vi "FPGA_init_FTL.vi"(6 "queue FPGA IN":refnum<queue>, 7 "FPGA VI Reference in":refnum<k20>, 8 "error in":errorcluster, 10 "variant":variant, 11 "Measuring QPD":bool) -> (0 "error out":errorcluster, 4 "queue FPGA OUT":refnum<queue>, 5 "FPGA VI Reference Out":refnum<k20>)   [LabVIEW 2015]
uses:
  CONTROLS/Q_FPGA_element.ctl
  <vilib>/FPGAPlugInAG/Dynamic/niLvFpga_Reset_Dynamic.vi
  <vilib>/FPGAPlugInAG/Dynamic/niLvFpga_Close_Dynamic.vi
  <vilib>/FPGAPlugInAG/PCIe-7841R/niLvFpga_Open_PCIe-7841R.vi
  <vilib>/rvi/interface/common/dynamic/niFpgaDynamicAddResources.vi
  <vilib>/Utility/error.llb/Error Cluster From Error Code.vi
  <vilib>/rvi/errors/niLvFpgaAdjustHostInterfaceError.vi
  <vilib>/FPGAPlugInAG/Dynamic/niLvFpga_Run_Dynamic.vi
  GLOBAL/Global_FPGA.vi
  <vilib>/rvi/interface/nirviMethod/nirviMethod.xnode
  <vilib>/rvi/interface/nirviCloseFPGA/nirviCloseFPGA.xnode
  <vilib>/rvi/interface/nirviOpenFPGA/nirviOpenFPGA.xnode
  FPGA/FPGA Bitfiles/FPGAv0_FPGATarget_FPGAtriggercamer_zs8MuLZc0ko.lvbitx
  <vilib>/rvi/interface/nirviReadWriteControl/nirviReadWriteControl.xnode
  NiFpgaLv.dll
  <vilib>/rvi/interface/Simulation/niFpgaSimulationCallBeginRW.vi
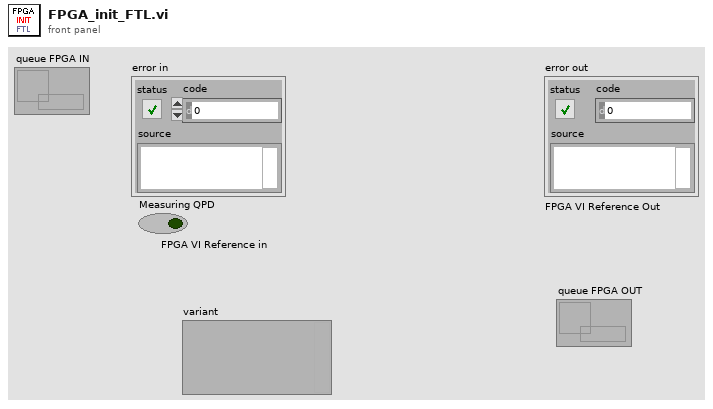
[diagram p1: front panel]
types:
  T1 = typedef "Q_FPGA_element.ctl" = cluster{"variant":variant, "Instruction":enum16{"FPGA_idle", "FPGA_initialize", "FPGA_error", "FPGA_security_stop", "FPGA_laser", "FPGA_start_stop_measure_QPD", "FPGA_measure_QPD", "FPGA_measure_QPD_noise", "FPGA_change_QPD_display", "FPGA_stop_measure_QPD", "FPGA_init_autofocus", "FPGA_init_single_scan", "FPGA_stop_single_scan", "FPGA_init_TL", "FPGA_close_TL", "FPGA_measure_QPD_FTL", "FPGA_init_FTL", "FPGA_init_single_scan_FTL", "FPGA_close_FTL", "FPGA_stop"}}
  T2 = cluster{"N laser lines":i32, "N Z positions":i32, "Laser lines":i32[], "Laser power":sgl[]}
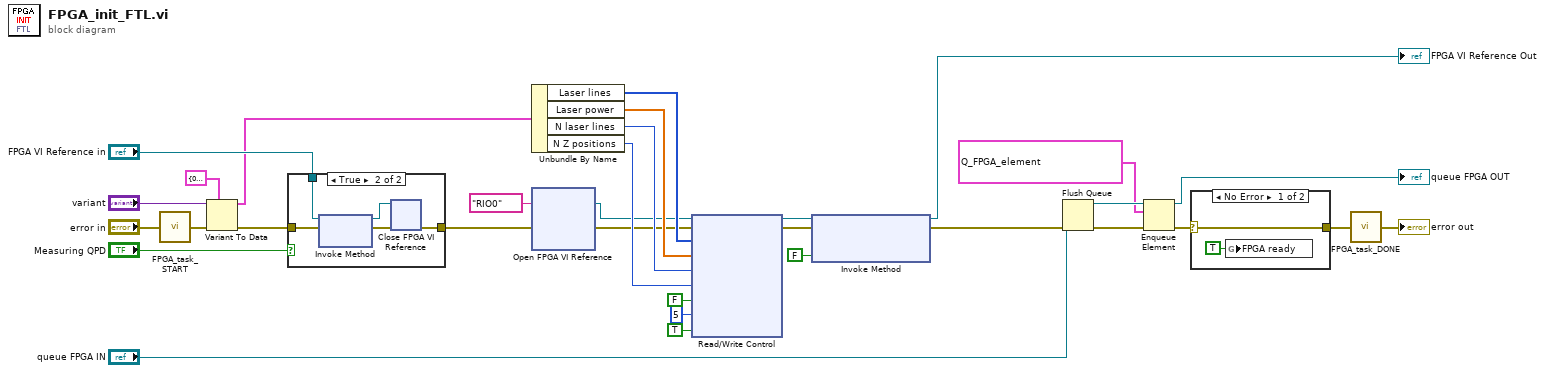
[diagram p0: block diagram]
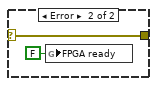
[diagram p3: hidden frame]
diagram:
  n1 = call "FPGA_task_START.vi"("error in"="error in") -> ("error out"=w20:errorcluster)
  n2 = Variant To Data(error in=w20, type=T2 {"N laser lines"=0, "N Z positions"=0, "Laser lines"=[0, 0, 0, 0, 0], "Laser power"=[0.0, 0.0, 0.0, 0.0, 0.0]} ("FPGA cluster"), Variant="variant") -> (data=w12:T2, error out=w21:errorcluster)
  n3 = case shown="True" "Measuring QPD" {
    tunnel: w21 -> [w33 w38]
    tunnel: "FPGA VI Reference in" -> [_ w37]
    tunnel: [w33 w34] -> w15
    frame False {
    }
    frame True {
      n4 = xnode "Invoke Method"("FPGA VI Reference In"=w37, "error in"=w38) -> ("FPGA VI Reference Out"=w35:refnum<k20>, "error out"=w36:errorcluster)
      n5 = xnode "Close FPGA VI Reference"("FPGA VI Reference In"=w35, "error in"=w36) -> ("error out"=w34:errorcluster)
    }
  }
  n6 = Unbundle By Name(w12) -> ("Laser lines"=w29:i32[], "Laser power"=w30:sgl[], "N laser lines"=w31:i32, "N Z positions"=w32:i32)
  n7 = xnode "Open FPGA VI Reference"("error in"=w15, "resource name"=tag "RIO0") -> ("FPGA VI Reference Out"=w25:refnum<k20>, "error out"=w24:errorcluster)
  n8 = xnode "Read/Write Control"("FPGA VI Reference In"=w25, "error in"=w24, "Laser lines"=w29, "Laser power"=w30, "N laser lines"=w31, "N Z positions"=w32, "stop"=FALSE, "Count(uSec)"=u32 5, "Reset counter"=TRUE) -> ("FPGA VI Reference Out"=w26:refnum<k20>, "error out"=w27:errorcluster)
  n9 = xnode "Invoke Method"("FPGA VI Reference In"=w26, "error in"=w27, "Wait Until Done (F)"=FALSE) -> ("FPGA VI Reference Out"=→"FPGA VI Reference Out":refnum<k20>, "error out"=w4:errorcluster)
  n10 = Flush Queue(queue="queue FPGA IN", error in (no error)=w4) -> (queue out=w7:refnum<queue>, error out=w6:errorcluster)  [unwired: 1 out]
  n11 = Enqueue Element(queue=w7, element=T1 {"variant"=variant, "Instruction"=enum."FPGA_measure_QPD_FTL"}, error in (no error)=w6) -> (queue out=→"queue FPGA OUT":refnum<queue>, error out=w1:errorcluster)  [unwired: 1 in, 1 out]
  n12 = case shown="No Error" w1 {
    selector: w1 -> [w39 w41]
    tunnel: [w39 w41] -> w14
    frame No Error {
      n13 = global write "Global_FPGA.vi" "FPGA ready"(TRUE ("FPGA ready")) -> ()
    }
    frame Error {
      n14 = global write "Global_FPGA.vi" "FPGA ready"(FALSE ("FPGA ready")) -> ()
    }
  }
  n15 = call "FPGA_task_DONE.vi"("error in"=w14) -> ("error out"=→"error out":errorcluster)
